vi "DIOSwitch.vi"(8 "error in":errorcluster, 9 "DIO Cluster":refnum<vi>, 10 "DIO Booleans New":T1, 11 "DIO Booleans Old":T1) -> (0 "error out":errorcluster)   [LabVIEW 2013]
uses:
  Controls/DIO Buttons.ctl
  <vilib>/DAQmx/write.llb/DAQmx Write (Digital Bool 1Line 1Point).vi
  <vilib>/DAQmx/create/channels.llb/DAQmx Create Channel (DO-Digital Output).vi
  <vilib>/DAQmx/miscellaneous.llb/DAQmx Fill In Error Info.vi
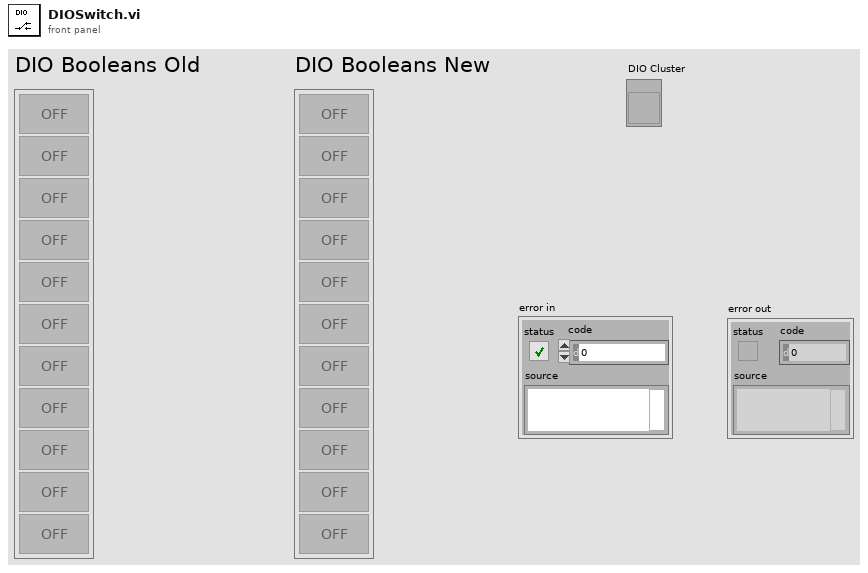
[diagram p1: front panel]
types:
  T1 = typedef "DIO Buttons.ctl" = bool[]
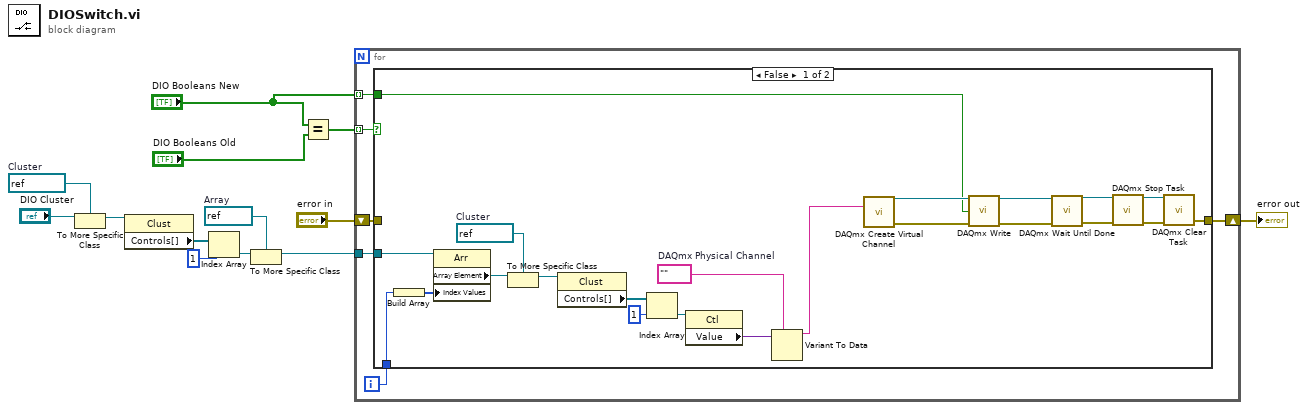
[diagram p0: block diagram]
diagram:
  w5 = refnum<vi> refnum  # Array
  w10 = refnum<vi> refnum  # Cluster
  n1 = To More Specific Class(target class=w10, reference="DIO Cluster") -> (specific class reference=w9:refnum<vi>)  [unwired: 1 in, 1 out]
  n2 = property class="Clust"(reference=w9) -> ("Controls[]"=w8:refnum<vi>[])  [unwired: 1 in, 2 out]
  n3 = Index Array(array=w8, index=1) -> (element=w6:refnum<vi>)
  n4 = To More Specific Class(target class=w5, reference=w6) -> (specific class reference=w4:refnum<vi>)  [unwired: 1 in, 1 out]
  n5 = Equal?(x="DIO Booleans New", y="DIO Booleans Old") -> (x = y?=w13:T1)
  n6 = for {
    tunnel: w13 -> [w19] mode=indexing
    tunnel: w4 -> [w18]
    tunnel: "DIO Booleans New" -> [w16] mode=indexing
    shift-right: [w15] -> w2
    shift-left: "error in" -> [w14]
    i -> [w17]
    n7 = case shown="False" w19 {
      tunnel: w18 -> [w41 _]
      tunnel: w17 -> [w40 _]
      tunnel: w16 -> [w21 _]
      tunnel: [w20 w42] -> w15
      tunnel: w14 -> [_ w42]
      frame False {
        w30 = tag ""  # DAQmx Physical Channel
        w37 = refnum<vi> refnum  # Cluster
        n8 = Build Array(w40) -> (w39:i32[])
        n9 = property class="Arr"(reference=w41, "Index Values"=w39) -> ("Array Element"=w38:refnum<vi>)  [unwired: 1 in, 2 out]
        n10 = To More Specific Class(target class=w37, reference=w38) -> (specific class reference=w36:refnum<vi>)  [unwired: 1 in, 1 out]
        n11 = property class="Clust"(reference=w36) -> ("Controls[]"=w35:refnum<vi>[])  [unwired: 1 in, 2 out]
        n12 = Index Array(array=w35, index=1) -> (element=w33:refnum<vi>)
        n13 = property class="Ctl"(reference=w33) -> ("Value"=w32:variant)  [unwired: 1 in, 2 out]
        n14 = Variant To Data(type=w30, Variant=w32) -> (data=w31:tag)  [unwired: 1 in, 1 out]
        n15 = call-poly <vilib>:"DAQmx Create Virtual Channel.vi"("lines"=w31) -> ("task out"=w22:refnum<k21>, "error out"=w23:errorcluster)  [unwired: 13 in]
        n16 = call-poly <vilib>:"DAQmx Write.vi"("task/channels in"=w22, "data"=w21, "error in"=w23) -> ("task out"=w25:refnum<k21>, "error out"=w24:errorcluster)  [unwired: 10 in, 1 out]
        n17 = call <vilib>:"DAQmx Wait Until Done.vi"("task/channels in"=w25, "error in"=w24) -> ("task out"=w27:refnum<k21>, "error out"=w26:errorcluster)  [unwired: 12 in]
        n18 = call <vilib>:"DAQmx Stop Task.vi"("task/channels in"=w27, "error in"=w26) -> ("task out"=w29:refnum<k21>, "error out"=w28:errorcluster)  [unwired: 12 in]
        n19 = call <vilib>:"DAQmx Clear Task.vi"("task in"=w29, "error in"=w28) -> ("error out"=w20:errorcluster)  [unwired: 13 in]
      }
      frame True {
      }
    }
  }
  "error out" <- w2
